vi "Step Function.vi"(1 "x":dbl format="%0.2f") -> (0 "step(x)":dbl format="%0.2f")   [LabVIEW 2024, in "NI_Gmath.lvlib"]
doc: "<p>Generates the step function for any real number <strong>x</strong>.</p>"
uses:
  NI_Gmath.lvlib
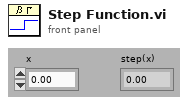
[diagram p1: front panel]
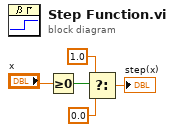
[diagram p0: block diagram]
diagram:
  n1 = Greater Or Equal To 0?(x="x") -> (x >= 0?=w4:bool)
  n2 = Select(t=1.0, s=w4, f=0.0) -> (s? t:f=→"step(x)":dbl)
